vi "czysc wykresy.vi"(8 "error in (no error)":errorcluster, 11 "Graphs Array":refnum<vi>[](array[refnum])) -> (0 "error out":errorcluster)   [LabVIEW 2014]
doc: "Czyœci wszystkie wykresy przy wyjœciu z programu"
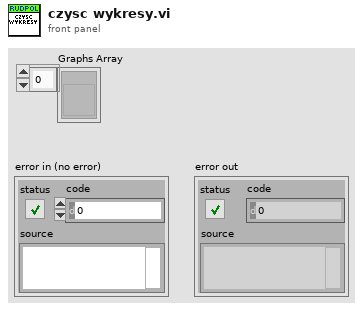
[diagram p1: front panel]
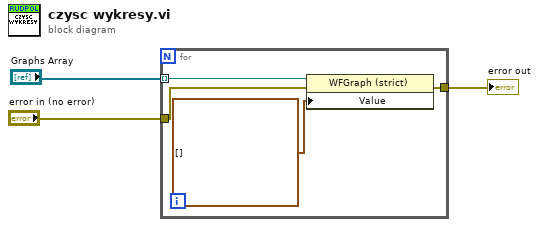
[diagram p0: block diagram]
diagram:
  n1 = for {
    tunnel: "Graphs Array" -> [w7] mode=indexing
    tunnel: [w5] -> w1
    tunnel: "error in (no error)" -> [w4]
    n2 = property class="WFGraph (strict)"(reference=w7, error in=w4, "Value"=waveform(dbl)[] []) -> (error out=w5:errorcluster)  [unwired: 1 out]
  }
  "error out" <- w1
